vi "MTMount_getNextSample_AzimuthDrives.vi"(8 "error in (no error)":errorcluster, 11 "Azimuth_Drives_Ctl":T1) -> (0 "error out":errorcluster, 2 "function return":i32, 3 "Azimuth_Drives_Ctl out":T1)   [LabVIEW 2018, in "SALLV_MTMount.lvlib"]
doc: "int MTMount_shm_getNextSample_Azimuth_DrivesLV(MTMount_Azimuth_DrivesLV *Azimuth_Drives_Ctl );"
uses:
  SALLV_MTMount.lvlib
  DataTypes/Azimuth_Drives.ctl
  SALLV_MTMount.so
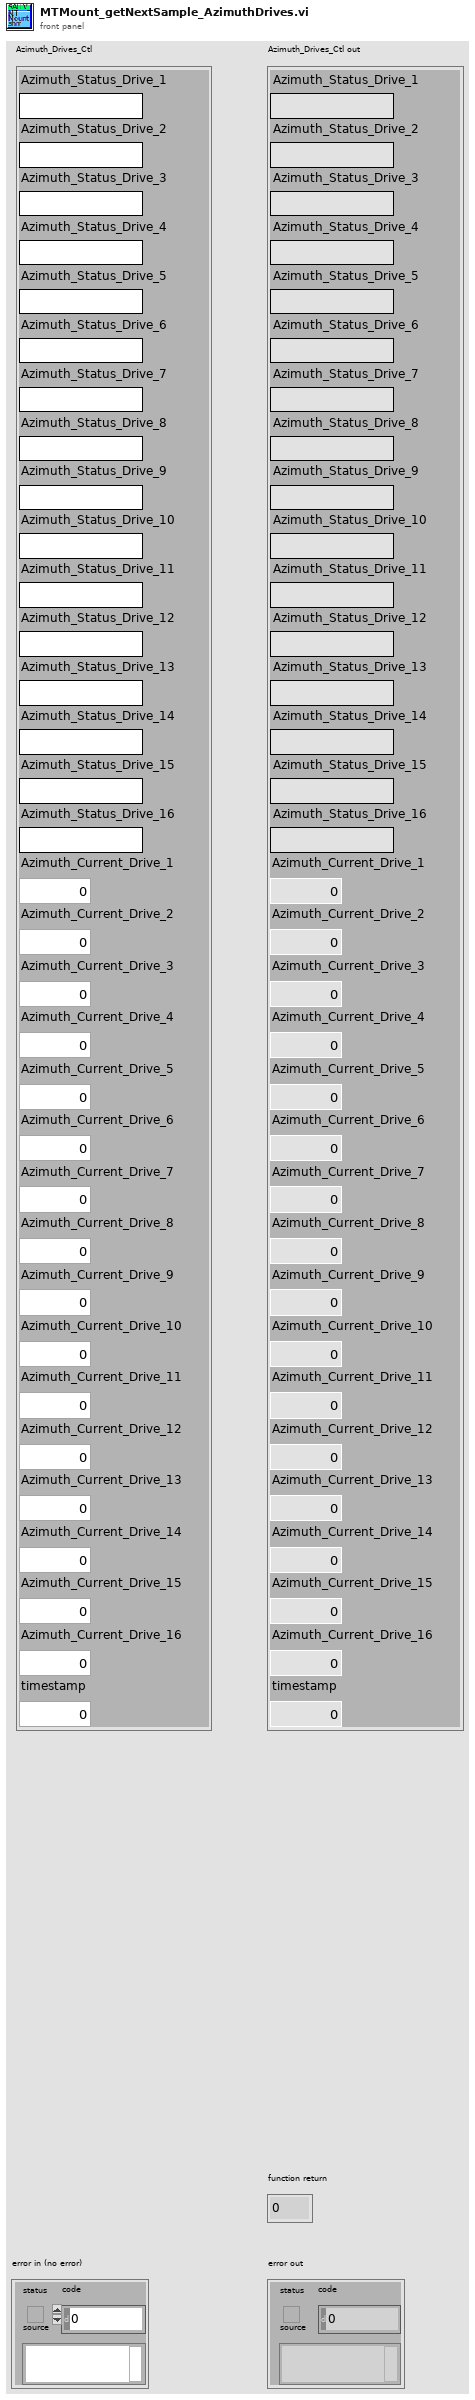
[diagram p1: front panel]
types:
  T1 = typedef "SALLV_MTMount.lvlib/Azimuth_Drives.ctl" = cluster{"Azimuth_Status_Drive_1":string, "Azimuth_Status_Drive_2":string, "Azimuth_Status_Drive_3":string, "Azimuth_Status_Drive_4":string, "Azimuth_Status_Drive_5":string, "Azimuth_Status_Drive_6":string, "Azimuth_Status_Drive_7":string, "Azimuth_Status_Drive_8":string, "Azimuth_Status_Drive_9":string, "Azimuth_Status_Drive_10":string, "Azimuth_Status_Drive_11":string, "Azimuth_Status_Drive_12":string, "Azimuth_Status_Drive_13":string, "Azimuth_Status_Drive_14":string, "Azimuth_Status_Drive_15":string, "Azimuth_Status_Drive_16":string, "Azimuth_Current_Drive_1":dbl, "Azimuth_Current_Drive_2":dbl, "Azimuth_Current_Drive_3":dbl, "Azimuth_Current_Drive_4":dbl, "Azimuth_Current_Drive_5":dbl, "Azimuth_Current_Drive_6":dbl, "Azimuth_Current_Drive_7":dbl, "Azimuth_Current_Drive_8":dbl, "Azimuth_Current_Drive_9":dbl, "Azimuth_Current_Drive_10":dbl, "Azimuth_Current_Drive_11":dbl, "Azimuth_Current_Drive_12":dbl, "Azimuth_Current_Drive_13":dbl, "Azimuth_Current_Drive_14":dbl, "Azimuth_Current_Drive_15":dbl, "Azimuth_Current_Drive_16":dbl, "timestamp":dbl}
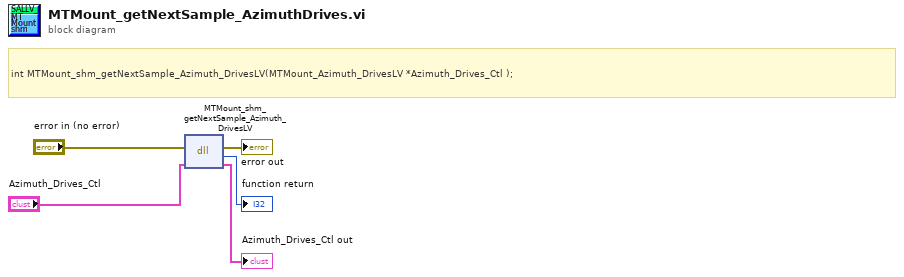
[diagram p0: block diagram]
diagram:
  # "int MTMount_shm_getNextSample_Azimuth_DrivesLV(MTMount_Azimuth_DrivesLV *Azimuth_Drives_Ctl );"
  n1 = dll-call lib="home/ttsai/Document/salApiMTMount/SALLV_MTMount/SALLV_MTMount.*" fn="MTMount_shm_getNextSample_Azimuth_DrivesLV"(error in="error in (no error)", "Azimuth_Drives_Ctl"="Azimuth_Drives_Ctl") -> (error out=→"error out":errorcluster, →"function return":i32, "Azimuth_Drives_Ctl"=→"Azimuth_Drives_Ctl out":T1)  [unwired: 2 in, 1 out]
